vi "Polynomial_Plot.vi"() -> ()   [LabVIEW 2022 SP3]
panel:
  in  "Xi":dbl
  in  "Number of \nData Points":dbl
  in  "C":dbl
  in  "B":dbl
  in  "A":dbl
  out "Y = A*x**2 + B*x + C":dbl[](graph)
  # "Polynomial Plot:\nEnter values for A, B, and C in the equation y = Ax**2 + Bx + C to see the plot of the function. Additionally, select the number of data points to be plotted as well as the starting value of x."
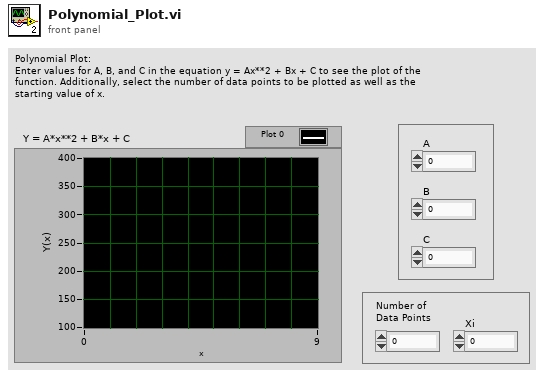
[diagram p1: front panel]
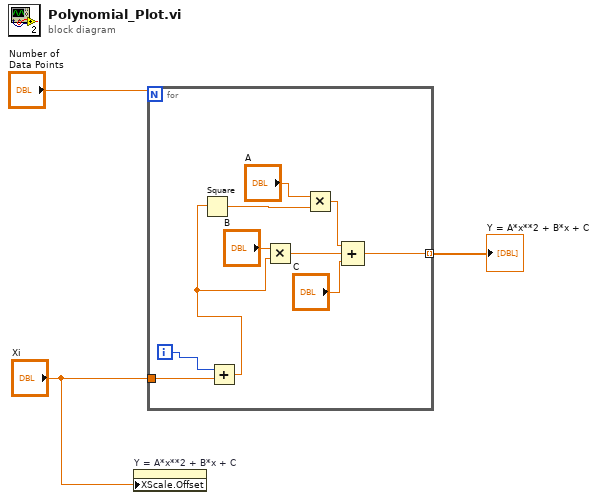
[diagram p0: block diagram]
diagram:
  n1 = property on="Y = A*x**2 + B*x + C" class="WFGraph (strict)"("XScale.Offset"="Xi") -> ()  [unwired: 2 in, 2 out]
  n2 = for {
    N: "Number of \nData Points" -> [_]
    tunnel: [w5] -> w2 mode=indexing
    tunnel: "Xi" -> [w4]
    i -> [w7]
    n3 = Add(x=w7, y=w4) -> (x+y=w6:dbl)
    n4 = Square(x=w6) -> (x^2=w13:dbl)
    n5 = Multiply(x="B", y=w6) -> (x*y=w10:dbl)
    n6 = Multiply(x="A", y=w13) -> (x*y=w9:dbl)
    n7 = Compound Arithmetic op=ADD(w9, w10, "C") -> (w5:dbl)
  }
  "Y = A*x**2 + B*x + C" <- w2
